vi "close 24C.vi"   [LabVIEW 2019]
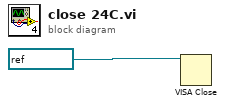
[diagram p0: block diagram]
diagram:
  n1 = VISA Close(VISA resource name=refnum<visa-resource-name> "COM3") -> ()  [unwired: 1 in, 1 out]
